vi "Byte Buffer.Read (Pointer).vi"(7 "bytes to copy":i32, 8 "error in (no error)":errorcluster, 9 "dst pointer":u64, 10 "buffer offset":i32, 11 "buffer in":string) -> (0 "error out":errorcluster, 3 "buffer out":string)   [LabVIEW 2016, in "VeriStand Data.lvlib"]
doc: "Reads data of size <B>bytes to copy</B> from the provided <B>buffer</B> at location <B>buffer offset</B> into the memory location specified by <B>dst pointer</B>."
uses:
  VeriStand Data.lvlib
  Memory Management/Memory Management.Handle Return.vi
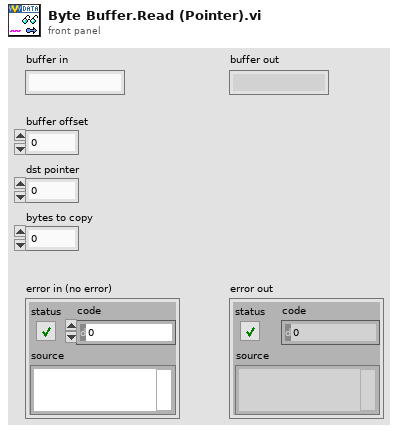
[diagram p1: front panel]
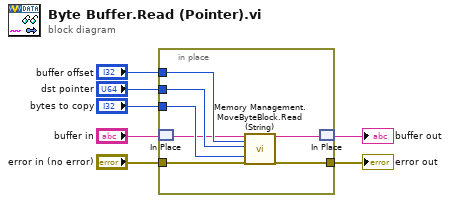
[diagram p0: block diagram]
diagram:
  n1 = in-place {
    in-place-border: "dst pointer" -> [w11]
    in-place-border: "buffer offset" -> [w12]
    in-place-border: "bytes to copy" -> [w10]
    in-place-border: "error in (no error)" -> [w14]
    in-place-border: [w13] -> w1
    n2 = in-place-match #1("buffer in") -> (w9:string)
    n3 = call "Memory Management.MoveByteBlock.Read (String).vi"("src in"=w9, "src offset (0)"=w12, "dst ptr in"=w11, "size"=w10, "error in (no error)"=w14) -> ("src out"=w8:string, "error out"=w13:errorcluster)  [unwired: 9 in, 4 out]
    n4 = in-place-match #1(w8) -> (→"buffer out":string)
  }
  "error out" <- w1
